vi "arduino sensirion read with retry (sub-vi).vi"(7 "max retries (2)":i32=2, 8 "error in (no error)":errorcluster, 9 "expected num sensors (12)":i32=12, 10 "read byte count (512)":u32=512, 11 "VISA resource name":refnum<visa-resource-name>) -> (0 "error out":errorcluster, 1 "relative timestamp":dbl, 2 "sensor data array":T1[](array[typedef]) {"temperature" scale=293.15..303.15 scale format="%#_3g"}, 3 "VISA resource name out":refnum<visa-resource-name>, 4 "retry count":i32)   [LabVIEW 2021]
uses:
  controls/sensirion_flow_sensor_data.ctl
  type-defs/ardruino_sensirion_read_states.ctl
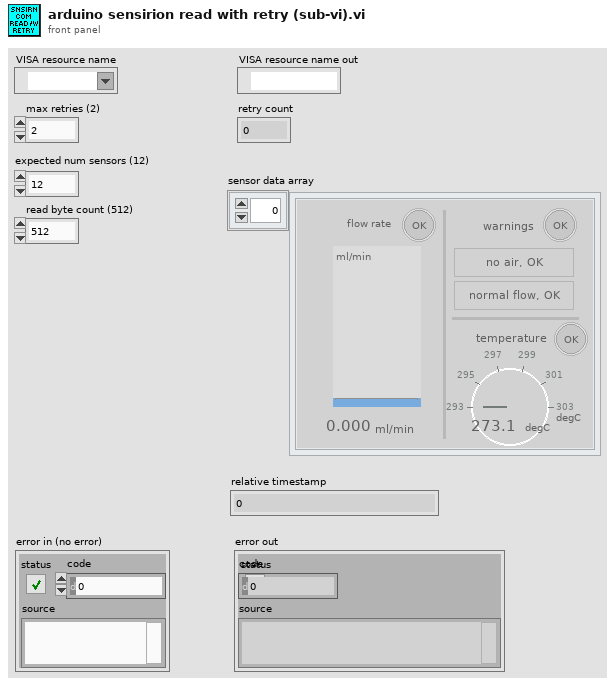
[diagram p1: front panel]
types:
  T1 = typedef "sensirion_flow_sensor_data.ctl" = cluster{"flow rate \n":dbl[unit], "flow val. status":bool, "temperature":dbl[unit], "temp. val status":bool, "air in line?":bool, "high flow?":bool, "flag. val status":bool}
  T2 = typedef "ardruino_sensirion_read_states.ctl" = enum16{"Initialize", "Read Buffer", "Retry", "Exit (Success)", "Fail", "Idle"}
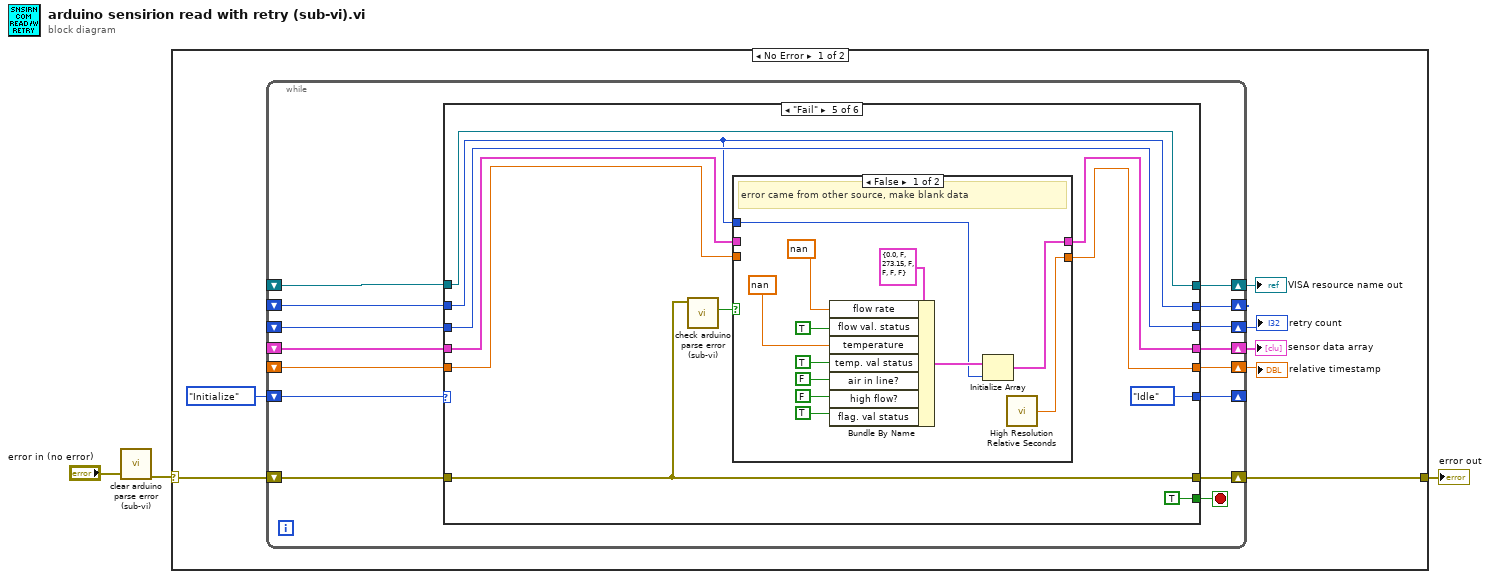
[diagram p0: block diagram]
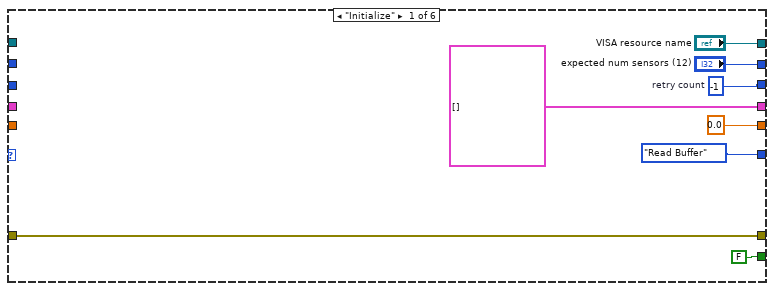
[diagram p2: hidden frame]
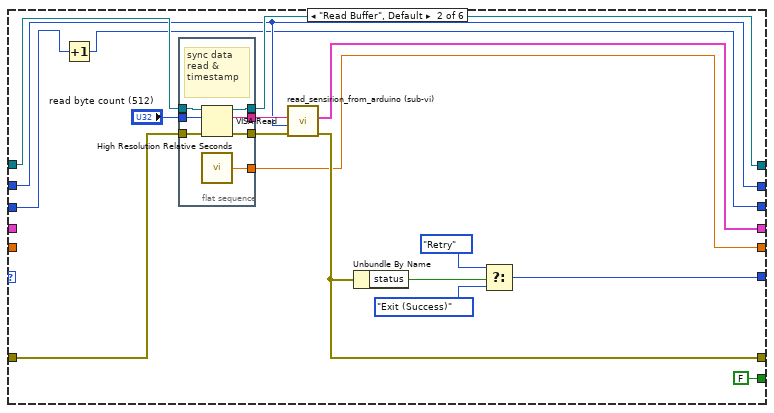
[diagram p3: hidden frame]
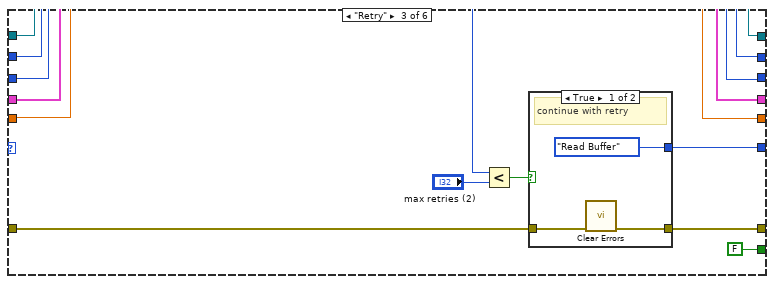
[diagram p4: hidden frame]
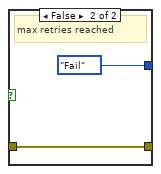
[diagram p5: hidden frame]
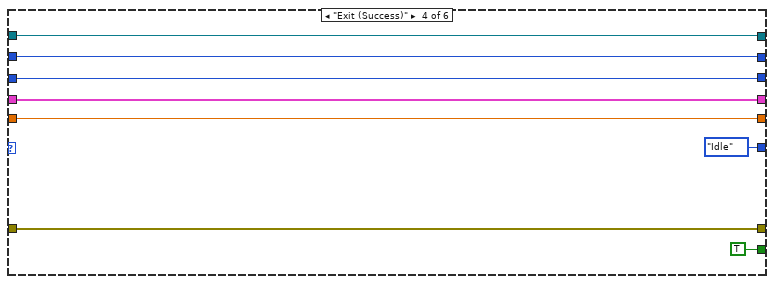
[diagram p6: hidden frame]
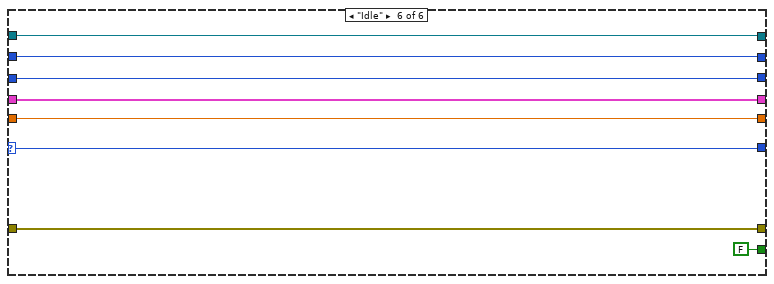
[diagram p8: hidden frame]
diagram:
  n1 = call "clear arduino parse error (sub-vi).vi"("error in"="error in (no error)") -> ("error out"=w1:errorcluster)  [unwired: 10 in]
  n2 = case shown="No Error" w1 {
    selector: w1 -> [w10 w115]
    tunnel: [w9 w115] -> w3
    frame No Error {
      n3 = while {
        shift-right: [w24] -> w9
        shift-left: w10 -> [w25]
        shift-right: [w23] -> w8
        shift-left: _ -> [w22]
        shift-right: [w21] -> _
        shift-left: _ -> [w20]
        shift-right: [w19] -> w5
        shift-left: _ -> [w18]
        shift-right: [w17] -> w7
        shift-left: _ -> [w16]
        shift-right: [w13] -> _
        shift-left: ardruino_sensirion_read_states."Initialize" ("Enum") -> [w14]
        shift-right: [w12] -> w4
        shift-left: _ -> [w11]
        stop <- w15 stop-if-true
        n4 = case shown="\"Fail\"" w14 {
          selector: w14 -> [_ _ _ _ _ w110]
          tunnel: w25 -> [w28 w50 w65 w76 w85 w109]
          tunnel: ["VISA resource name" w47 w68 w79 w92 w114] -> w23
          tunnel: [w28 w43 w61 w76 w85 w109] -> w24
          tunnel: w22 -> [_ w45 w68 w79 w92 w114]
          tunnel: ["expected num sensors (12)" w44 w67 w78 w87 w113] -> w21
          tunnel: w20 -> [_ w44 w67 w78 w87 w113]
          tunnel: [w31 w37 w63 w77 w91 w112] -> w19
          tunnel: w18 -> [_ w36 w63 w77 w91 w112]
          tunnel: [T1[] [] ("sensor data array") w42 w66 w81 w88 w111] -> w17
          tunnel: w16 -> [_ _ w66 w81 w89 w111]
          tunnel: [FALSE FALSE FALSE TRUE TRUE FALSE] -> w15
          tunnel: [ardruino_sensirion_read_states."Read Buffer" ("Enum") w35 w59 ardruino_sensirion_read_states."Idle" ("Enum") ardruino_sensirion_read_states."Idle" ("Enum") w110] -> w13
          tunnel: [0.0 ("relative seconds") w34 w58 w74 w82 w107] -> w12
          tunnel: w11 -> [_ _ w58 w74 w83 w107]
          frame "Initialize" {
            w31 = -1  # retry count
          }
          frame "Read Buffer", Default {
            n5 = Increment(x=w36) -> (x+1=w37:i32)
            n6 = flat-sequence {
              tunnel: w50 -> [w57]
              tunnel: [w56] -> w49
              tunnel: [w55] -> w48
              tunnel: [w54] -> w47
              tunnel: "read byte count (512)" -> [w53]
              tunnel: w45 -> [w52]
              tunnel: [w51] -> w34
              frame #0 {
                # "sync data read & timestamp"
                n7 = VISA Read(VISA resource name=w52, byte count=w53, error in (no error)=w57) -> (VISA resource name out=w54:refnum<visa-resource-name>, read buffer=w55:string, error out=w56:errorcluster)  [unwired: 1 out]
                n8 = call <vilib>:"High Resolution Relative Seconds.vi"() -> ("relative seconds"=w51:dbl)
              }
            }
            n9 = call "read_sensirion_from_arduino (sub-vi).vi"("error in"=w49, "expected num sensors (12)"=w44, "serial buffer in"=w48) -> ("error out"=w43:errorcluster, "sensor data array"=w42:T1[])  [unwired: 7 in]
            n10 = Unbundle By Name(w43) -> ("status"=w41:bool)
            n11 = Select(t=ardruino_sensirion_read_states."Retry", s=w41, f=ardruino_sensirion_read_states."Exit (Success)" ("Enum")) -> (s? t:f=w35:T2)
          }
          frame "Retry" {
            n12 = Less?(x=w63, y="max retries (2)") -> (x < y?=w62:bool)
            n13 = case shown="True" w62 {
              tunnel: w65 -> [w70 w72]
              tunnel: [ardruino_sensirion_read_states."Read Buffer" ("Enum") ardruino_sensirion_read_states."Fail" ("Enum")] -> w59
              tunnel: [w69 w72] -> w61
              frame True {
                # "continue with retry"
                n14 = call <vilib>:"Clear Errors.vi"("error in (no error)"=w70) -> ("error out"=w69:errorcluster)  [unwired: 5 in, 1 out]
              }
              frame False {
                # "max retries reached"
              }
            }
          }
          frame "Exit (Success)" {
          }
          frame "Fail" {
            n15 = call "check arduino parse error (sub-vi).vi"("error"=w85) -> ("is arduino parse error?"=w84:bool)  [unwired: 10 in]
            n16 = case shown="False" w84 {
              tunnel: w89 -> [_ w106]
              tunnel: [w94 w106] -> w88
              tunnel: w87 -> [w95 _]
              tunnel: w83 -> [_ w105]
              tunnel: [w93 w105] -> w82
              frame False {
                # "error came from other source, make blank data"
                n17 = Bundle By Name(cluster=T1 {"flow rate \n"=0.0, "flow val. status"=FALSE, "temperature"=273.15, "temp. val status"=FALSE, "air in line?"=FALSE, "high flow?"=FALSE, "flag. val status"=FALSE} ("sensirion flow sensor data cluster"), "flow rate"=dbl[unit] nan, "flow val. status"=TRUE, "temperature"=dbl[unit] nan ("temp.\n(C)"), "temp. val status"=TRUE, "air in line?"=FALSE ("air in \nline?"), "high flow?"=FALSE ("high \nflow?"), "flag. val status"=TRUE) -> (w96:T1)
                n18 = Initialize Array(w96, w95) -> (w94:T1[])
                n19 = call <vilib>:"High Resolution Relative Seconds.vi"() -> ("relative seconds"=w93:dbl)
              }
              frame True {
                # "error came from arduino read, data is OK"
              }
            }
          }
          frame "Idle" {
          }
        }
      }
      "VISA resource name out" <- w8
      "sensor data array" <- w7
      "retry count" <- w5
      "relative timestamp" <- w4
    }
    frame Error {
    }
  }
  "error out" <- w3
